vi "Get Index by Serial.vi"(8 "error in (no error)":errorcluster, 10 "Serial Number":string, 11 "RTL-SDR in":refnum<class "RTL-SDR.lvclass">) -> (0 "error out":errorcluster, 2 "Index":i32, 3 "RTL-SDR out":refnum<class "RTL-SDR.lvclass">)   [LabVIEW 2015, in "RTL-SDR.lvclass"]
uses:
  RTL-SDR.lvclass
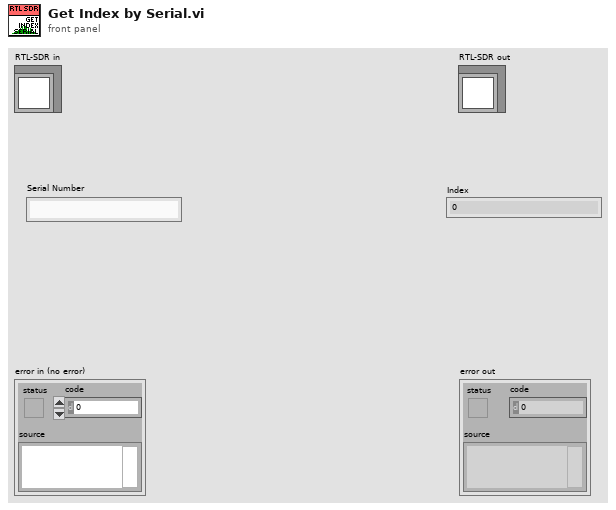
[diagram p1: front panel]
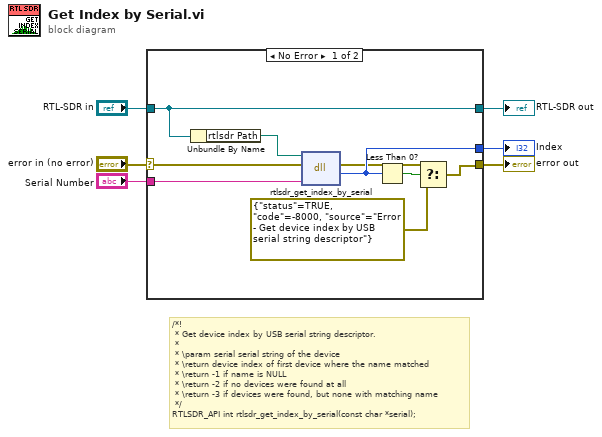
[diagram p0: block diagram]
diagram:
  # "/*!\n * Get device index by USB serial string descriptor.\n *\n * \\param serial serial string of the device\n * \\return device index of first device where the name matched\n * \\return -1 if name is NULL\n * \\return -2 if no devices were found at all\n * \\return -3 if devices were found, but none with matching name\n */\nRTLSDR_API int rtlsdr_get_index_by_serial(const char *serial);"
  n1 = case shown="No Error" "error in (no error)" {
    selector: "error in (no error)" -> [w15 w17]
    tunnel: [w7 w17] -> w5
    tunnel: [w14 w16] -> w3
    tunnel: "RTL-SDR in" -> [w14 w16]
    tunnel: "Serial Number" -> [w12 _]
    tunnel: [w9 _] -> w1
    frame No Error {
      n2 = Unbundle By Name(w14) -> ("rtlsdr Path"=w13:path)
      n3 = dll-call lib="C:/Users/Ivan/Desktop/D-23-09-24 (RTL-SDR)/Project (Pelleng-SDR)/RTL-SDR Class/dll/rtlsdr.*" fn="rtlsdr_get_index_by_serial"(path in=w13, error in=w15, "serial"=w12) -> (error out=w8:errorcluster, "return type"=w9:i32)  [unwired: 2 in, 1 out]
      n4 = Less Than 0?(x=w9) -> (x < 0?=w10:bool)
      n5 = Select(t=w8, s=w10, f=errorcluster {"status"=TRUE, "code"=-8000, "source"="Error - Get device index by USB serial string descriptor"} ("error out")) -> (s? t:f=w7:errorcluster)
    }
    frame Error {
    }
  }
  "error out" <- w5
  "RTL-SDR out" <- w3
  "Index" <- w1
